vi "Max_Lobe.vi"(9 "Beta Mean":dbl, 10 "Alpha Mean":dbl, 11 "Theta Mean":dbl) -> (1 "Beta":bool, 2 "Alpha":bool, 3 "Theta":bool)   [LabVIEW 2019]
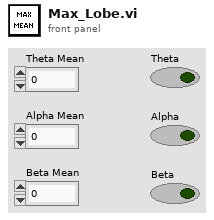
[diagram p1: front panel]
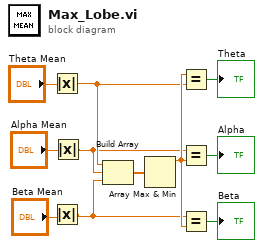
[diagram p0: block diagram]
diagram:
  n1 = Absolute Value(x="Theta Mean") -> (abs(x)=w5:dbl)
  n2 = Absolute Value(x="Beta Mean") -> (abs(x)=w2:dbl)
  n3 = Absolute Value(x="Alpha Mean") -> (abs(x)=w1:dbl)
  n4 = Build Array(w5, w1, w2) -> (w7:dbl[])
  n5 = Array Max & Min(array=w7) -> (max value=w10:dbl)  [unwired: 3 out]
  n6 = Equal?(x=w10, y=w5) -> (x = y?=→"Theta":bool)
  n7 = Equal?(x=w1, y=w10) -> (x = y?=→"Alpha":bool)
  n8 = Equal?(x=w2, y=w10) -> (x = y?=→"Beta":bool)
